vi "Recipes Enqueue.vi"(7 "Opposite End?":bool, 8 "error in (no error)":errorcluster, 10 "Expansion Queue Element":T1, 11 "Queue in":refnum<queue>) -> (0 "error out":errorcluster, 3 "Queue out":refnum<queue>)   [LabVIEW 2017, in "Recipes.lvclass"]
uses:
  Recipes.lvclass
  Type Defs/Recipes Queue Element.ctl
  Type Defs/Recipes State.ctl
  Recipes.lvclass/Recipes.ctl
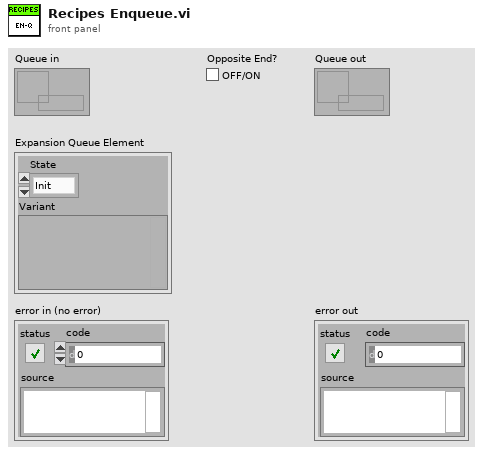
[diagram p1: front panel]
types:
  T1 = typedef "Recipes.lvclass/Recipes Queue Element.ctl" = cluster{"State":T2, "Variant":variant}
  T2 = typedef "Recipes.lvclass/Recipes State.ctl" = enum16{"Init", "Go", "Stop", "Idle", "Error", "Shutdown"}
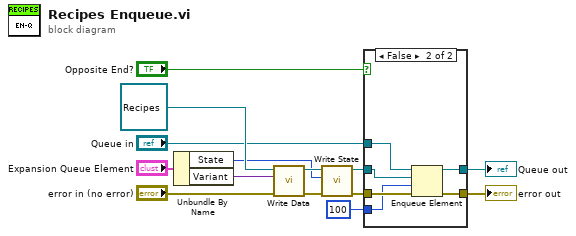
[diagram p0: block diagram]
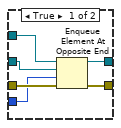
[diagram p2: hidden frame]
diagram:
  n1 = Unbundle By Name("Expansion Queue Element") -> ("State"=w9:T2, "Variant"=w8:variant)
  n2 = call "Write Data.vi"("error in (no error)"="error in (no error)", "Data"=w8, "Expansion in"=refnum<class "Recipes.lvclass"> refnum) -> ("error out"=w12:errorcluster, "Expansion out"=w13:refnum<class "Recipes.lvclass">)  [unwired: 7 in]
  n3 = call "Write State.vi"("error in (no error)"=w12, "State"=w9, "Expansion in"=w13) -> ("error out"=w4:errorcluster, "Expansion out"=w3:refnum<class "Recipes.lvclass">)  [unwired: 7 in]
  n4 = case shown="False" "Opposite End?" {
    tunnel: [w20 w26] -> w2
    tunnel: "Queue in" -> [w19 w25]
    tunnel: w3 -> [w18 w24]
    tunnel: w4 -> [w17 w23]
    tunnel: [w16 w22] -> w1
    tunnel: 100 ("timeout in ms (-1)") -> [w15 w21]
    frame True {
      n5 = Enqueue Element At Opposite End(queue=w19, element=w18, timeout in ms (-1)=w15, error in (no error)=w17) -> (queue out=w20:refnum<queue>, error out=w16:errorcluster)  [unwired: 1 out]
    }
    frame False {
      n6 = Enqueue Element(queue=w25, element=w24, timeout in ms (-1)=w21, error in (no error)=w23) -> (queue out=w26:refnum<queue>, error out=w22:errorcluster)  [unwired: 1 out]
    }
  }
  "error out" <- w1
  "Queue out" <- w2
